vi "(auto) Skip same balls(SubVI).vi"(10 "Circles Calibrated (Shape Detection 1)":T1(array[cluster]), 11 "balls counter":i32) -> (2 "balls coutnter Out":i32, 3 "arrOut":i32[](array[numeric]))   [LabVIEW 2017]
uses:
  <vilib>/imath/engines/lvmath2/RunTimeEngine/NodeEndStatement/NIMS_NodeEndStatement_Output.vi
  <instcachedir>/0/NIMS_NodeEndStatement_Output_53EC0D466D134D7ABD903AC30B43404B.lvgen/NIMS_NodeEndStatement_Output_53EC0D466D134D7ABD903AC30B43404B_012.vi
  <instcachedir>/0/NIMS_NodeEndStatement_Output_53EC0D466D134D7ABD903AC30B43404B.lvgen/NIMS_NodeEndStatement_Output_53EC0D466D134D7ABD903AC30B43404B_010.vi
  <vilib>/imath/engines/lvmath2/RunTimeEngine/ErrorHandling/NIMS_Finalize Error.vi
panel:
  in  "range":dbl
  out "y1":sgl
  out "x1":sgl
  out "y2":sgl
  out "x2":sgl
  out "indx":i32
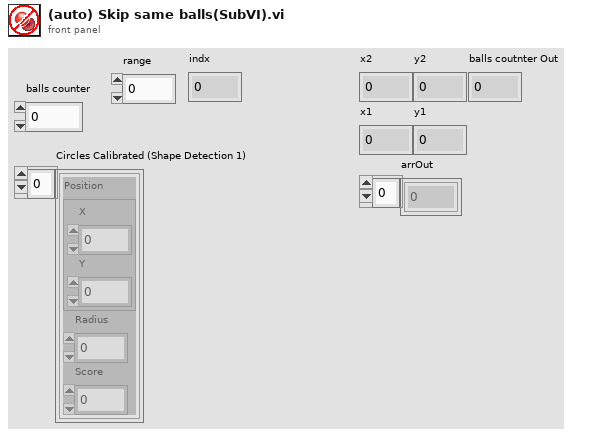
[diagram p1: front panel]
types:
  T1 = cluster{"Position":cluster{"X":sgl, "Y":sgl}, "Radius":dbl, "Score":dbl}[]
  T2 = cluster{"Position":cluster{"X":sgl, "Y":sgl}, "Radius":dbl, "Score":dbl}
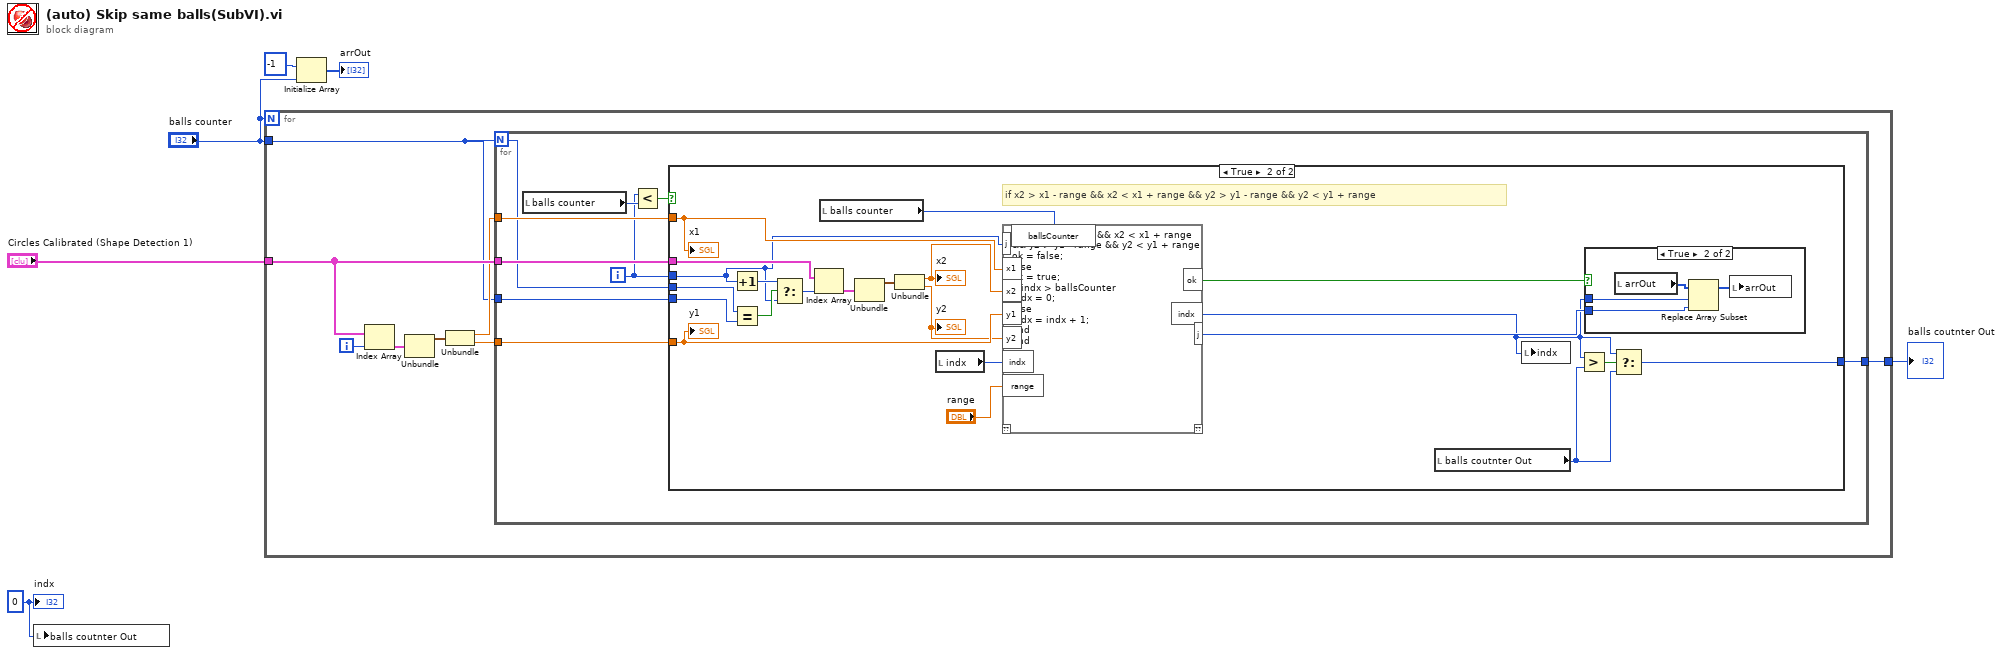
[diagram p0: block diagram]
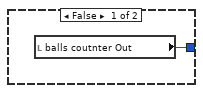
[diagram p2: hidden frame]
diagram:
  w1 = 0 ("indx")
  n1 = local write "balls coutnter Out"(w1) -> ()
  n2 = for {
    N: "balls counter" -> [_]
    tunnel: "Circles Calibrated (Shape Detection 1)" -> [w11]
    tunnel: "balls counter" -> [w7]
    tunnel: [w8] -> w2
    i -> [w12]
    n3 = Index Array(array=w11, index=w12) -> (element=w14:T2)
    n4 = Unbundle(w14) -> ("Position"=w13:cluster{"X":sgl, "Y":sgl})  [unwired: 2 out]
    n5 = Unbundle(w13) -> ("X"=w10:sgl, "Y"=w9:sgl)
    n6 = for {
      N: w7 -> [w16]
      tunnel: w11 -> [w23]
      tunnel: w10 -> [w22]
      tunnel: w9 -> [w21]
      tunnel: [w19] -> w8
      tunnel: w7 -> [w20]
      i -> [w15]
      n7 = local read "balls counter"() -> (w18:i32)
      n8 = Less?(x=w15, y=w18) -> (x < y?=w17:bool)
      n9 = case shown="True" w17 {
        tunnel: w23 -> [_ w46]
        tunnel: w22 -> [_ w43]
        tunnel: w21 -> [_ w42]
        tunnel: w20 -> [_ w36]
        tunnel: w16 -> [_ w33]
        tunnel: w15 -> [_ w31]
        tunnel: [w24 w29] -> w19
        frame False {
          n10 = local read "balls coutnter Out"() -> (w24:i32)
        }
        frame True {
          # "if x2 > x1 - range && x2 < x1 + range && y2 > y1 - range && y2 < y1 + range"
          n11 = Increment(x=w31) -> (x+1=w34:i32)
          n12 = Equal?(x=w33, y=w36) -> (x = y?=w35:bool)
          n13 = Select(t=w34, s=w35, f=w31) -> (s? t:f=w32:i32)
          n14 = Index Array(array=w46, index=w32) -> (element=w45:T2)
          n15 = local read "balls counter"() -> (w25:i32)
          n16 = Unbundle(w45) -> ("Position"=w44:cluster{"X":sgl, "Y":sgl})  [unwired: 2 out]
          n17 = Unbundle(w44) -> ("X"=w41:sgl, "Y"=w40:sgl)
          "x2" <- w41
          "y2" <- w40
          n18 = local read "indx"() -> (w30:i32)
          n19 = mathscript code="if x2 > x1 - range && x2 < x1 + range && y2 > y1 - range && y2 < y1 + range\nok = false;\nelse\nok = true;\nif indx > ballsCounter\nindx = 0;\nelse\nindx = indx + 1;\nend\nend"("x1"=w43, "x2"=w41, "y1"=w42, "y2"=w40, "indx"=w30, "range"="range", "j"=w31, "ballsCounter"=w25) -> ("ok"=w38:bool, "indx"=w26:i32, "j"=w37:i32)  [unwired: 1 in, 1 out]
          n20 = local read "balls coutnter Out"() -> (w27:i32)
          n21 = local write "indx"(w26) -> ()
          n22 = Greater?(x=w26, y=w27) -> (0:w28:bool)
          n23 = case shown="True" w38 {
            tunnel: w26 -> [_ w48]
            tunnel: w37 -> [_ w47]
            frame False {
            }
            frame True {
              n24 = local read "arrOut"() -> (w49:i32[])
              n25 = Replace Array Subset(array=w49, new element=w47, index=w48) -> (w50:i32[])
              n26 = local write "arrOut"(w50) -> ()
            }
          }
          n27 = Select(t=w26, s=w28, f=w27) -> (s? t:f=w29:i32)
          "x1" <- w43
          "y1" <- w42
        }
      }
    }
  }
  "balls coutnter Out" <- w2
  n28 = Initialize Array(-1 ("element"), "balls counter") -> (→"arrOut":i32[])
  "indx" <- w1
